vi "ma_time continuity checker.vi"(0 "timestamp previous":timestamp, 5 "dt previous":dbl, 7 "timestamp current":timestamp, 9 "dt current":dbl, 11 "error in (no error)":errorcluster) -> (4 "epsilon used":dbl, 6 "t0 changed":bool, 10 "dt changed":bool, 15 "error out":errorcluster)   [LabVIEW 2022 SP3, in "NI_MABase.lvlib"]
uses:
  NI_MABase.lvlib
  ma_Compute t0 eps timestamp.vi
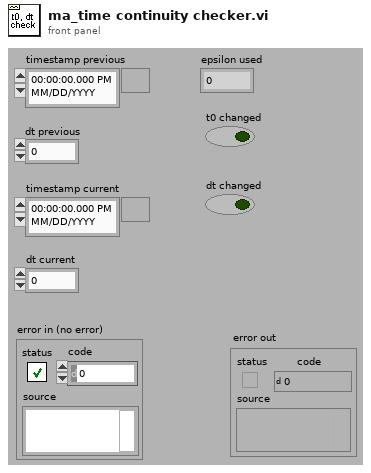
[diagram p1: front panel]
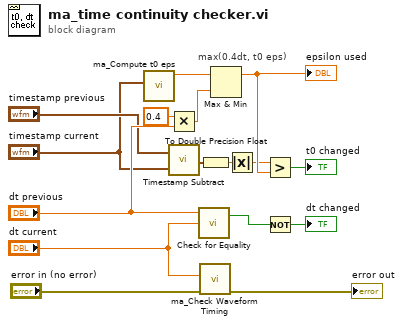
[diagram p0: block diagram]
diagram:
  # "max(0.4dt, t0 eps)"
  n1 = call-poly "ma_Compute t0 eps.vi"("t0 entry"="timestamp current") -> ("t0 eps"=w6:dbl)  [unwired: 10 in]
  n2 = Multiply(x=0.4, y="dt previous") -> (x*y=w8:dbl)
  n3 = call "Timestamp Subtract.vi"("y"="timestamp current", "x"="timestamp previous") -> ("x - y"=w15:timestamp)
  n4 = call "Check for Equality.vi"("n2"="dt current", "n1"="dt previous") -> ("equal?"=w11:bool)  [unwired: 1 in, 1 out]
  n5 = call "ma_Check Waveform Timing.vi"("error in (no error)"="error in (no error)", "dt"="dt current") -> ("error out"=→"error out":errorcluster)  [unwired: 8 in, 1 out]
  n6 = To Double Precision Float(number=w15) -> (double precision float=w16:dbl)
  n7 = Max & Min(x=w6, y=w8) -> (max(x,y)=w10:dbl)  [unwired: 1 out]
  "epsilon used" <- w10
  n8 = Absolute Value(x=w16) -> (abs(x)=w9:dbl)
  n9 = Greater?(x=w9, y=w10) -> (0:→"t0 changed":bool)
  n10 = Not(x=w11) -> (.not. x?=→"dt changed":bool)
